vi "WriteAndRead (SubVI).vi"(8 "error in (no error)":errorcluster, 10 "Write":string, 11 "VISA Refnum in":refnum<visa-resource-name>) -> (0 "error out":errorcluster, 3 "VISA resource name out":refnum<visa-resource-name>)   [LabVIEW 2020]
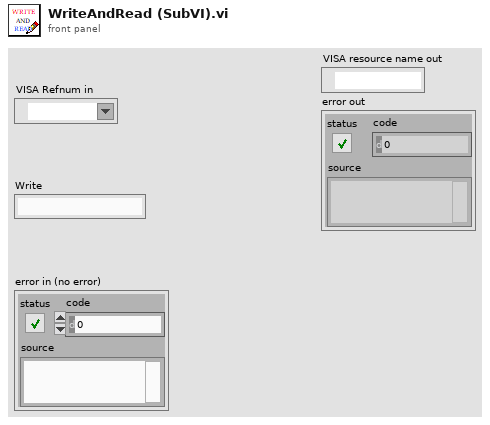
[diagram p1: front panel]
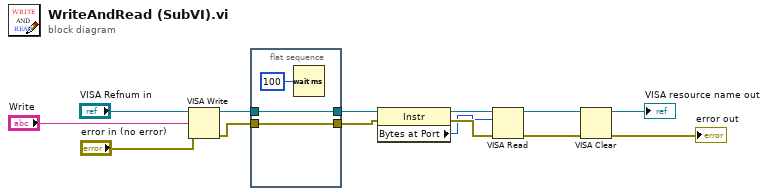
[diagram p0: block diagram]
diagram:
  n1 = VISA Write(VISA resource name="VISA Refnum in", write buffer="Write", error in (no error)="error in (no error)") -> (VISA resource name out=w3:refnum<visa-resource-name>, error out=w2:errorcluster)  [unwired: 1 out]
  n2 = flat-sequence {
    tunnel: [w16] -> w4
    tunnel: w3 -> [w16]
    tunnel: w2 -> [w15]
    tunnel: [w15] -> w1
    frame #0 {
      n3 = Wait (ms)(milliseconds to wait=u32 100) -> ()  [unwired: 1 out]
    }
  }
  n4 = property class="Instr"(reference=w4, error in=w1) -> (reference out=w9:refnum<visa-resource-name>, error out=w8:errorcluster, "Bytes at Port"=w7:u32)
  n5 = VISA Read(VISA resource name=w9, byte count=w7, error in (no error)=w8) -> (VISA resource name out=w5:refnum<visa-resource-name>, error out=w6:errorcluster)  [unwired: 2 out]
  n6 = VISA Clear(VISA resource name=w5, error in (no error)=w6) -> (VISA resource name out=→"VISA resource name out":refnum<visa-resource-name>, error out=→"error out":errorcluster)
